vi "WriteFeaturesToMap.vi"(8 "error in (no error)":errorcluster, 10 "Map in":T7, 11 "Group":T1) -> (0 "error out":errorcluster, 2 "Map out":T7, 3 "Group out":T1)   [LabVIEW 2017, in "McsaAnalysisHighRate.lvlib"]
uses:
  <vilib>/addons/InsightCM/Devices/Shared/Mcsa/McsaAnalysisHighRate/McsaAnalysisHighRate.lvlib
  <vilib>/addons/PointValueMap/controls/PointMap.ctl
  <vilib>/addons/InsightCM/Devices/Shared/Mcsa/McsaAnalysisHighRate/controls/Group.ctl
  <vilib>/addons/InsightCM/Utilities/Analysis/MCSA/controls/McsaChannel.ctl
  <vilib>/addons/InsightCM/Utilities/Analysis/Shared/controls/Feature.ctl
  <vilib>/addons/InsightCM/Utilities/Analysis/Shared/controls/AmplitudeScale.ctl
  <vilib>/addons/InsightCM/MessageBus/Base/controls/KeyValuePair.ctl
  <vilib>/addons/InsightCM/Utilities/Analysis/MCSA/controls/McsaMotor.ctl
  <vilib>/addons/PointValueMap/subVIs/Point_Write_double.vi
  <vilib>/addons/PointValueMap/PointValueMap.lvlib
  <vilib>/addons/InsightCM/Utilities/Analysis/Shared/AnalysisHelper.lvlib
  <vilib>/addons/InsightCM/Utilities/Analysis/MCSA/McsaAnalysisFunctions.lvlib
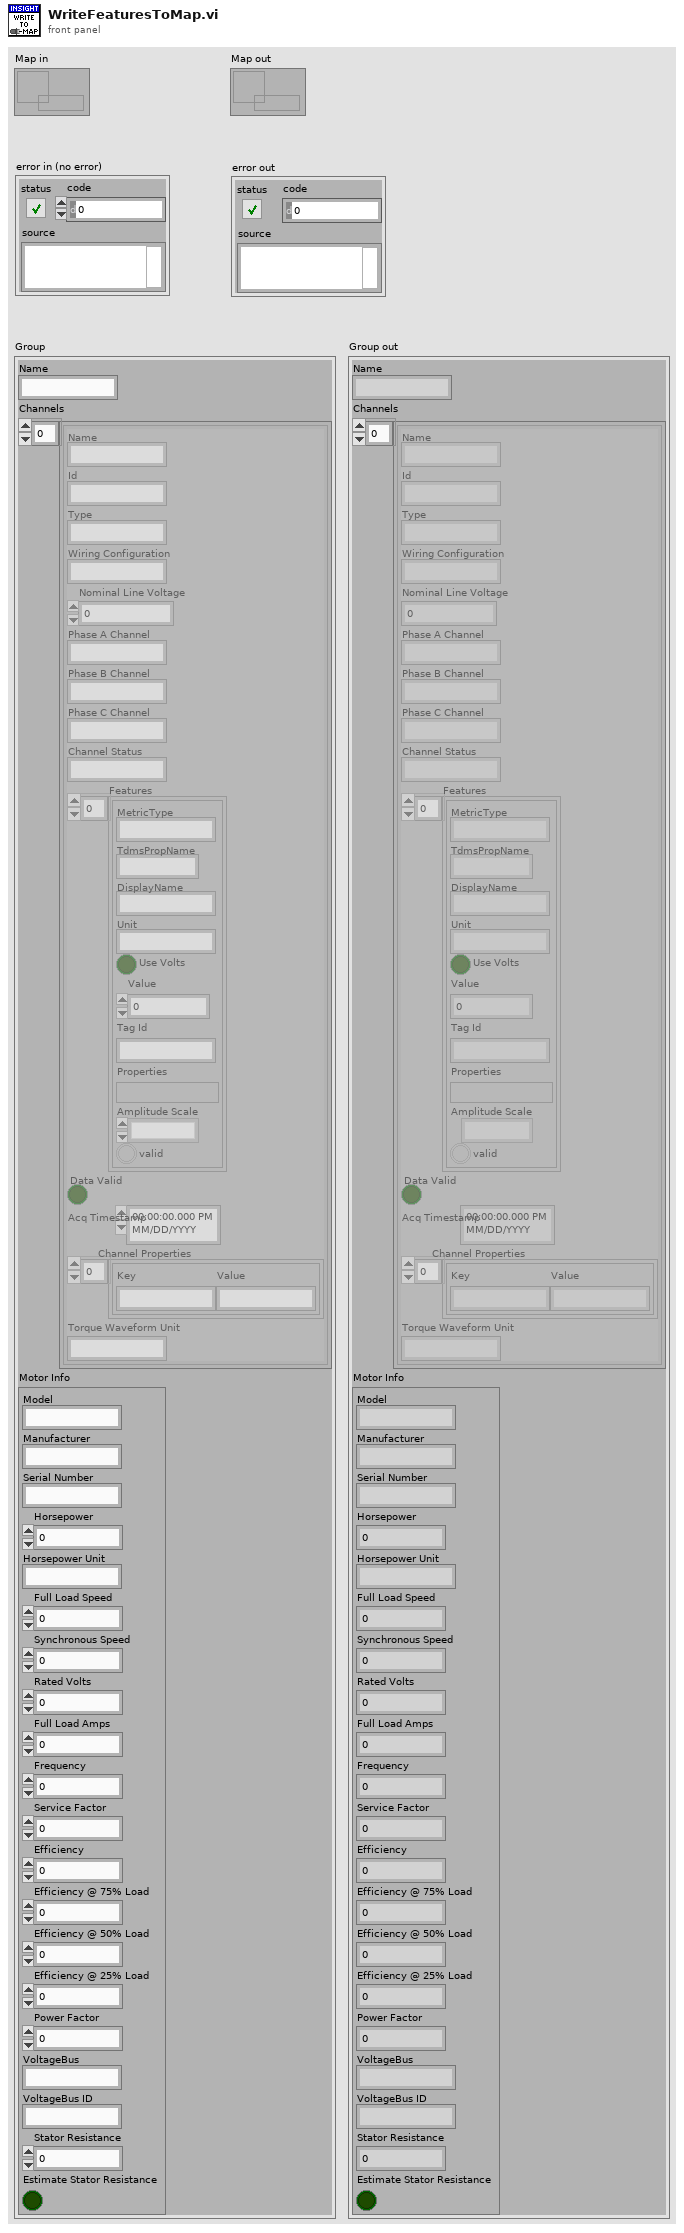
[diagram p1: front panel]
types:
  T1 = typedef "McsaAnalysisHighRate.lvlib/Group.ctl" = cluster{"Name":string, "Channels":T2[], "Motor Info":T6}
  T2 = typedef "McsaAnalysisFunctions.lvlib/McsaChannel.ctl" = cluster{"Name":string, "Id":string, "Type":string, "Wiring Configuration":string, "Nominal Line Voltage":dbl, "Phase A Channel":string, "Phase B Channel":string, "Phase C Channel":string, "Channel Status":string, "Features":T3[], "Data Valid":bool, "Acq Timestamp":timestamp, "Channel Properties":T5[], "Torque Waveform Unit":string}
  T3 = typedef "AnalysisHelper.lvlib/Feature.ctl" = cluster{"MetricType":string, "TdmsPropName":string, "DisplayName":string, "Unit":string, "Use Volts":bool, "Value":dbl, "Tag Id":string, "Properties":variant, "Amplitude Scale":T4, "valid":bool}
  T4 = typedef "AnalysisHelper.lvlib/AmplitudeScale.ctl" = enum16{"rms", "peak", "pk-pk"}
  T5 = typedef "KeyValuePair.ctl" = cluster{"Key":string, "Value":string}
  T6 = typedef "McsaAnalysisFunctions.lvlib/McsaMotor.ctl" = cluster{"Model":string, "Manufacturer":string, "Serial Number":string, "Horsepower":dbl, "Horsepower Unit":string, "Full Load Speed":dbl, "Synchronous Speed":dbl, "Rated Volts":dbl, "Full Load Amps":dbl, "Frequency":dbl, "Service Factor":dbl, "Efficiency":dbl, "Efficiency @ 75% Load":dbl, "Efficiency @ 50% Load":dbl, "Efficiency @ 25% Load":dbl, "Power Factor":dbl, "VoltageBus":string, "VoltageBus ID":string, "Stator Resistance":dbl, "Estimate Stator Resistance":bool}
  T7 = typedef "PointValueMap.lvlib/PointMap.ctl" = refnum<data-value>
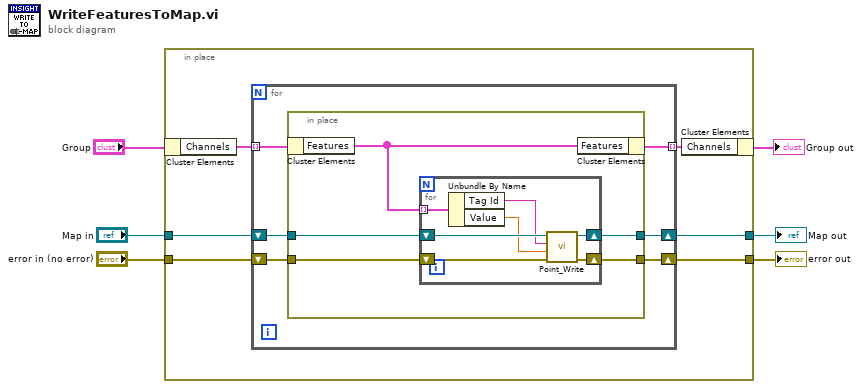
[diagram p0: block diagram]
diagram:
  n1 = in-place {
    in-place-border: "Map in" -> [w12]
    in-place-border: "error in (no error)" -> [w11]
    in-place-border: [w7] -> w6
    in-place-border: [w10] -> w3
    n2 = in-place-cluster #1("Group") -> ("Channels"=w9:T2[])
    n3 = for {
      tunnel: w9 -> [w18] mode=indexing
      shift-right: [w14] -> w10
      shift-left: w12 -> [w17]
      tunnel: [w13] -> w8 mode=indexing
      shift-right: [w15] -> w7
      shift-left: w11 -> [w16]
      n4 = in-place {
        in-place-border: w17 -> [w23]
        in-place-border: w16 -> [w22]
        in-place-border: [w19] -> w15
        in-place-border: [w21] -> w14
        n5 = in-place-cluster #2(w18) -> ("Features"=w20:T3[])
        n6 = for {
          tunnel: w20 -> [w30] mode=indexing
          shift-right: [w25] -> w21
          shift-left: w23 -> [w29]
          shift-right: [w24] -> w19
          shift-left: w22 -> [w28]
          n7 = Unbundle By Name(w30) -> ("Tag Id"=w26:string, "Value"=w27:dbl)
          n8 = call-poly <vilib>:"Point_Write.vi"("Error In"=w28, "Value"=w27, "Tag"=w26, "Map"=w29) -> ("Error Out"=w24:errorcluster, "Map Out"=w25:T7)  [unwired: 6 in]
        }
        n9 = in-place-cluster #2("Features"=w20) -> (w13:T2)
      }
    }
    n10 = in-place-cluster #1("Channels"=w8) -> (→"Group out":T1)
  }
  "error out" <- w6
  "Map out" <- w3
